vi "电导率电极校准.vi"() -> ()   [LabVIEW 2016, in "斯坦道多参数.lvlib"]
uses:
  <vilib>/Utility/miscctls.llb/LVPointTypeDef.ctl
  <vilib>/Analysis/NI_AALBase.lvlib
  <vilib>/ptbypt/NI_PtbyPt.lvlib
panel:
  in  "刷新按钮":bool
  out "第二点信号值":dbl
  out "第一点信号值":dbl
  out "通讯状态":string
  out "盐度":dbl caption="盐度测量值" format="%#.2f"
  out "温度":dbl format="%#.2f"
  out "当前信号值":dbl caption="信号值" format="%#.2f"
  in  "校准停止":bool
  in  "校准启动":bool
  out "波形图表":dbl(graph) caption="历史曲线"
  out "第二点校准值":dbl
  out "第一点校准值":dbl
  in  "校准模式":enum16{"两点校准", "单点校准"}(ring)=enum."单点校准"
  out "提示":string
  out "最小值":sgl format="%#.2f"
  out "最大值":sgl format="%#.2f"
  out "mean":dbl caption="均值" format="%#.2f"
  out "standard deviation":dbl caption="标准差" format="%#.2f"
  out "变异系数":dbl format="%#.6f"
  out "标液2":dbl
  out "标液1":dbl
  out "当前读取值":dbl caption="测量值" format="%#.2f"
  out "电极系数":dbl format="%#.6f"
  out "偏移值补偿":dbl caption="电导率偏移修正值" format="%#.2f"
  out "温度补偿系数":dbl format="%#.6f"
  # "电导率电极设定"
  # "ppt"
  # "请选择校准模式:"
  # "℃"
  # "μS/cm"
  # "cm"
  # "-1"
  # "%"
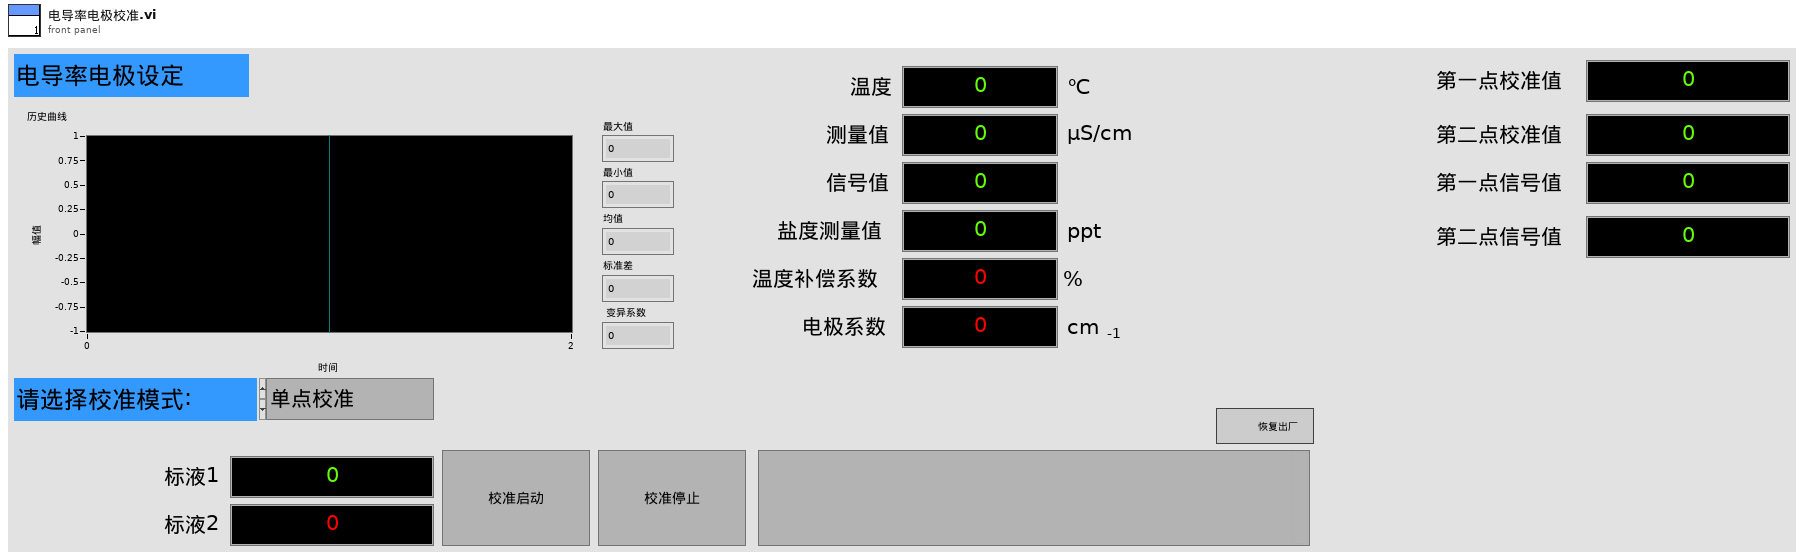
[diagram p1: front panel]
types:
  T1 = typedef "LVPointTypeDef.ctl" = cluster{"Horizontal":i16, "Vertical":i16}
  T2 = cluster{"电极状态标志":u16, "电极型号标志":u16, "电导率测量值":sgl, "温度测量值":sgl, "电导率信号值":sgl, "温度信号值":sgl, "温度补偿系数":sgl, "电导率偏移修正值":sgl, "温度偏移修正值":sgl, "手动温度补偿值":sgl, "电导率电极零点":sgl, "电导率电极斜率":sgl, "命令滤波设定":u16, "温度模式":enum16{"ATC", "MTC"}, "生产批次":u16, "电极序号":u16, "串口地址":u16, "串口波特率":enum16{"9600", "19200", "115200"}, "串口校验位":enum16{"NONE", "ODD", "EVEN"}, "串口停止位":enum16{"1bit", "2bit"}, "第一点标准值":sgl, "第二点标准值":sgl}
  T3 = enum8{"Enabled", "Disabled", "Disabled and Grayed Out"}
  T4 = cluster{"ph":bool, "DO":bool, "Cond":bool, "Turb":bool, "叶绿素a":bool, "藻密度":bool, "ORP":bool}
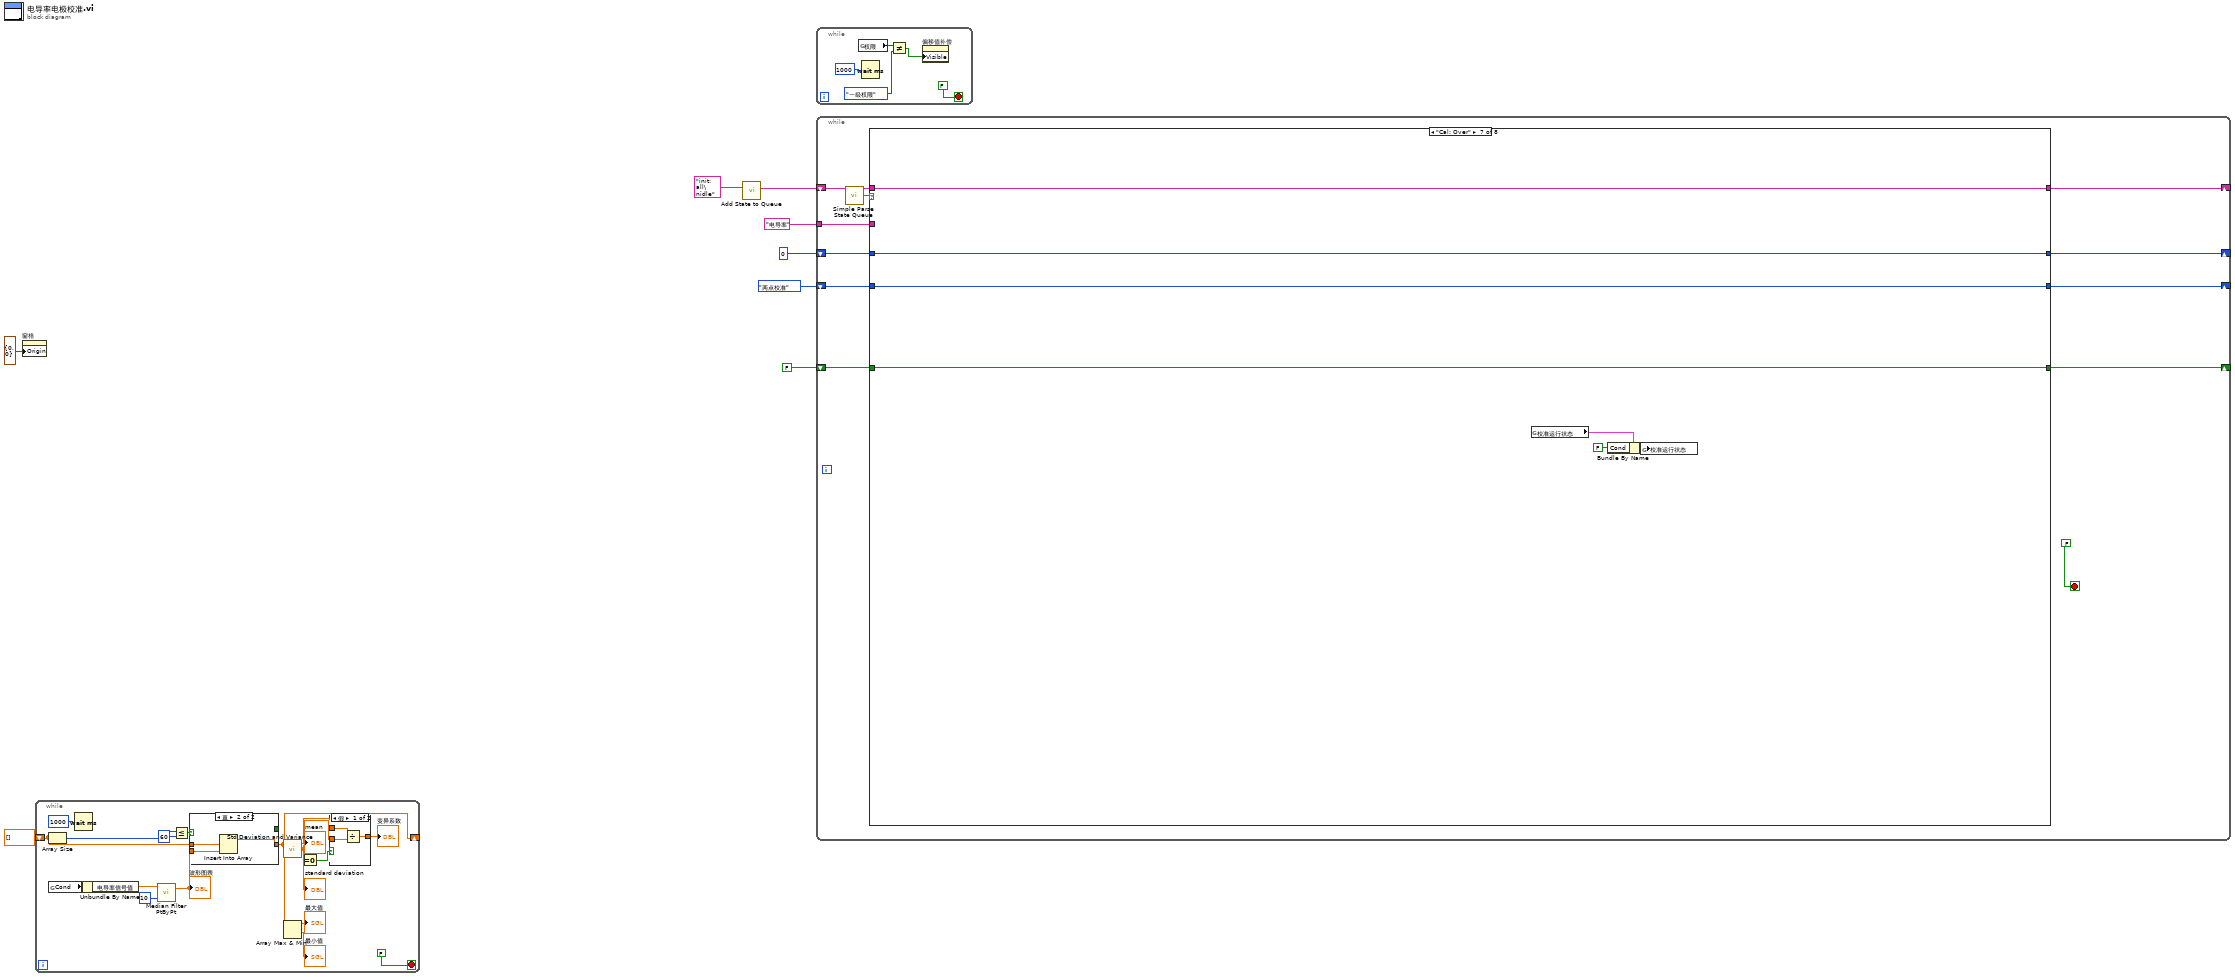
[diagram p0: block diagram]
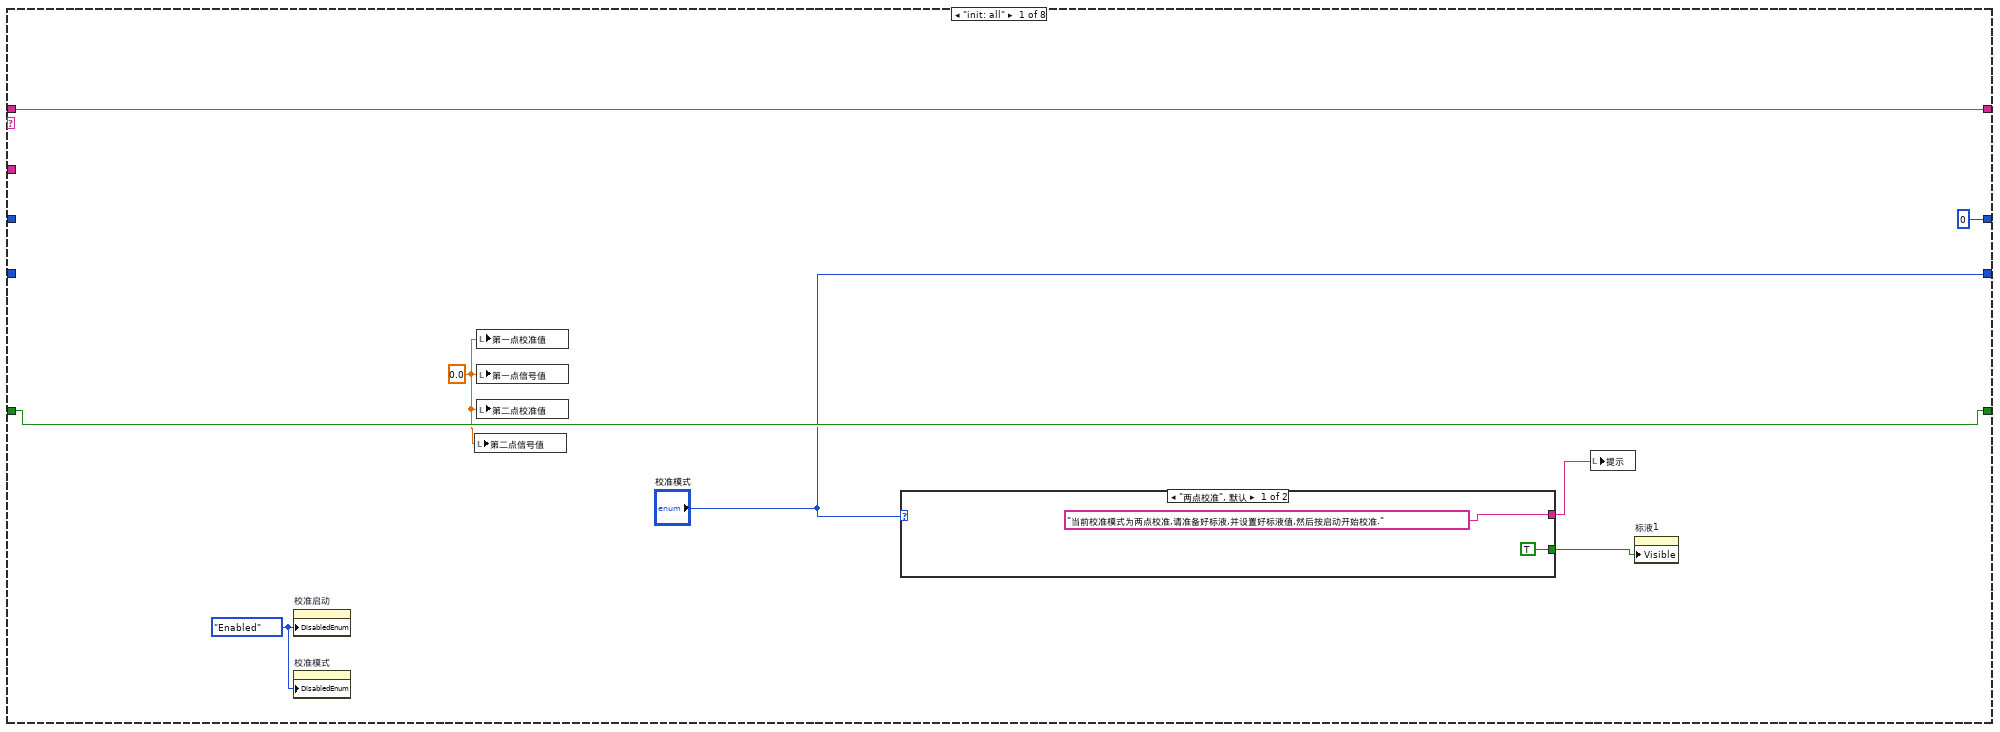
[diagram p2: hidden frame]
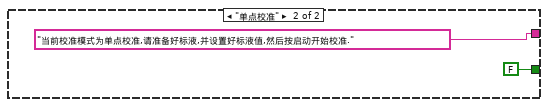
[diagram p3: hidden frame]
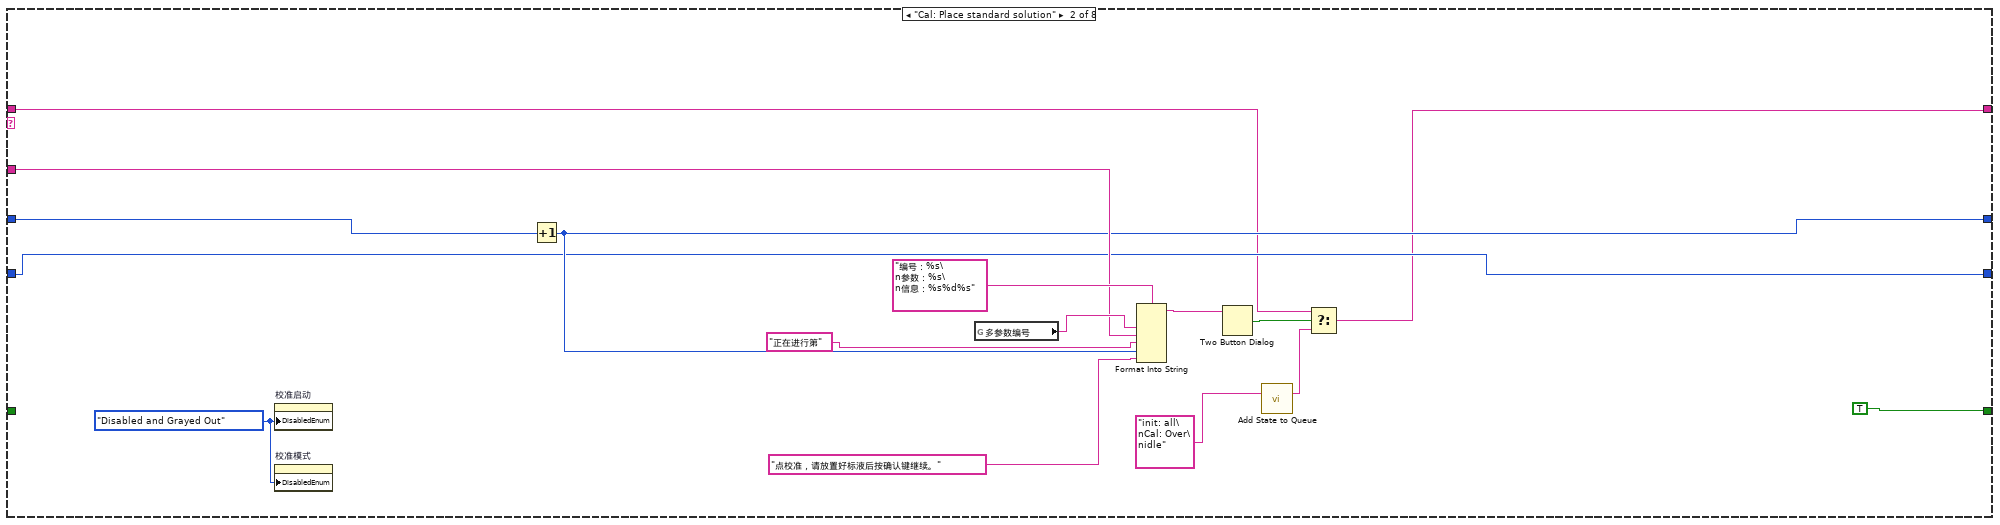
[diagram p4: hidden frame]
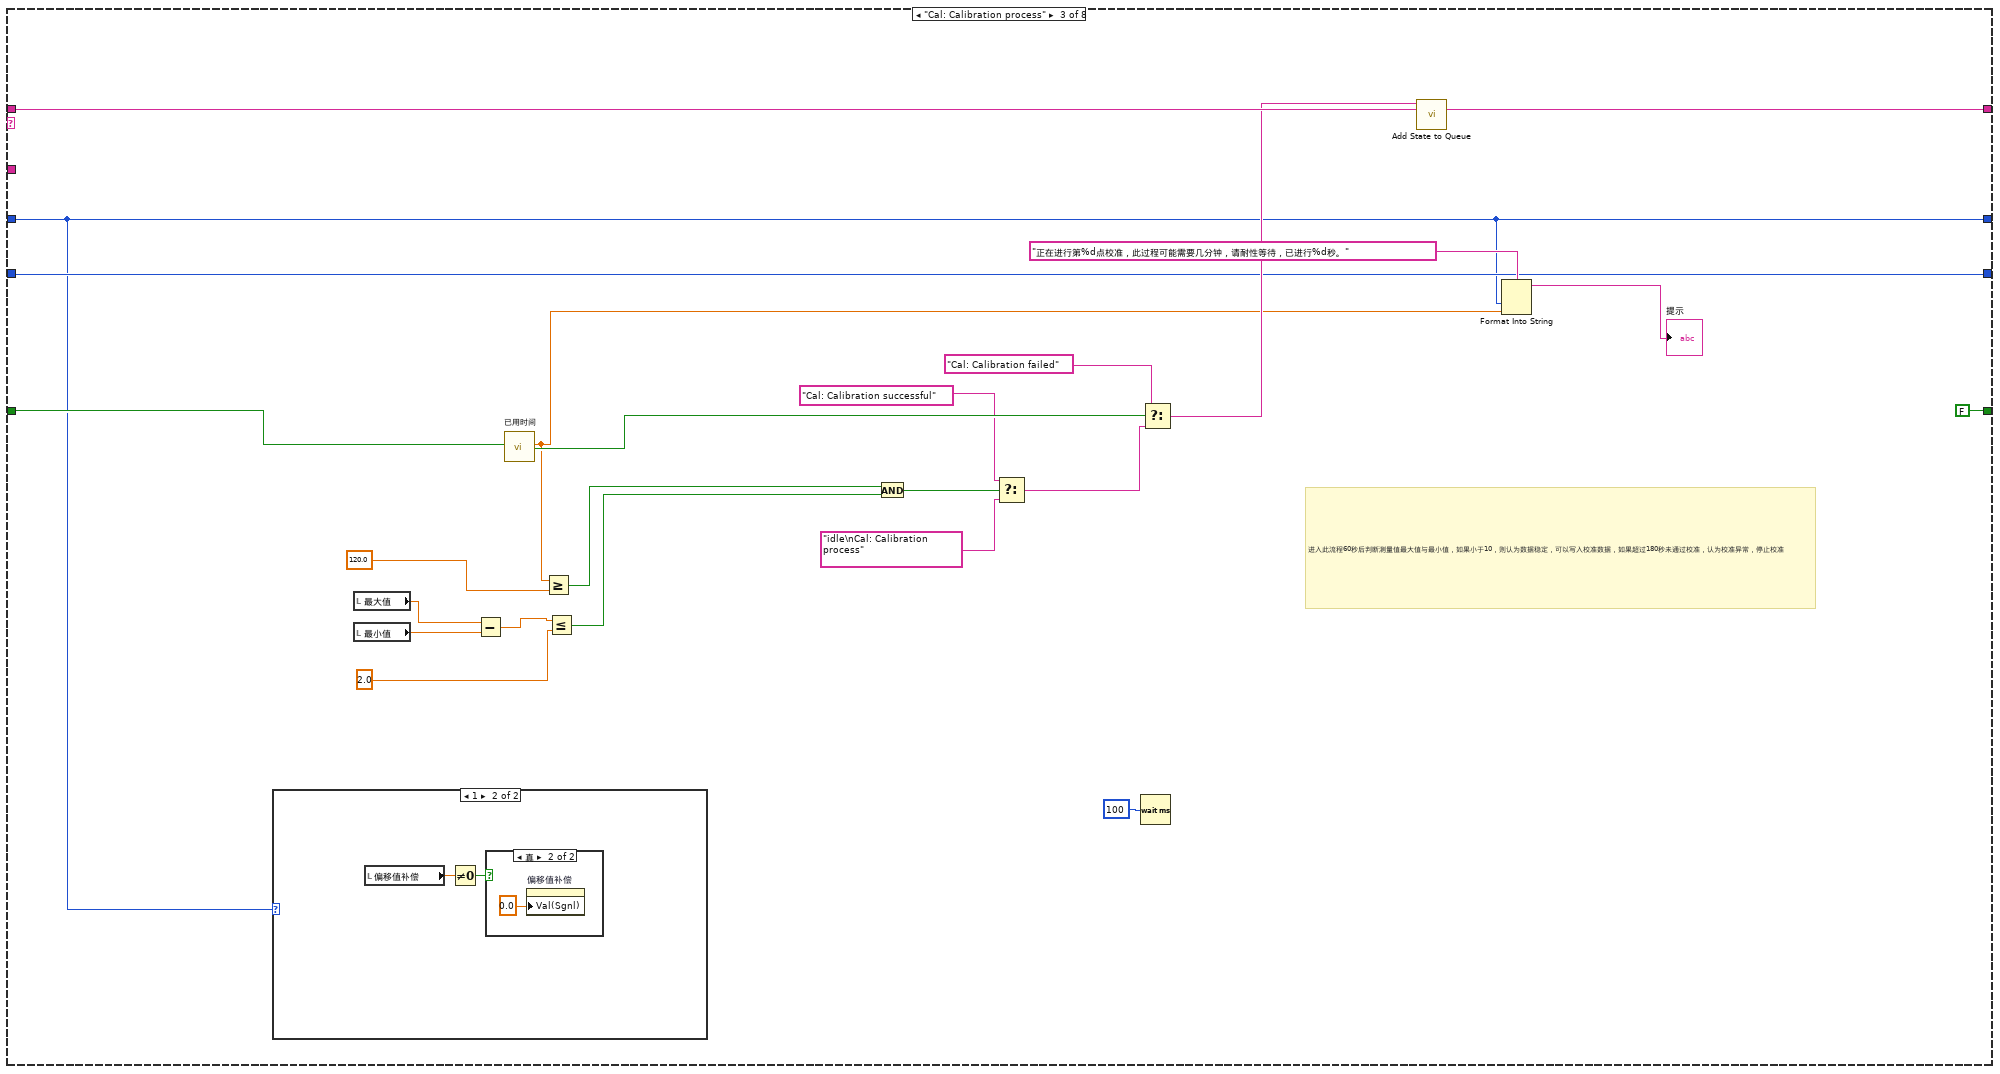
[diagram p5: hidden frame]
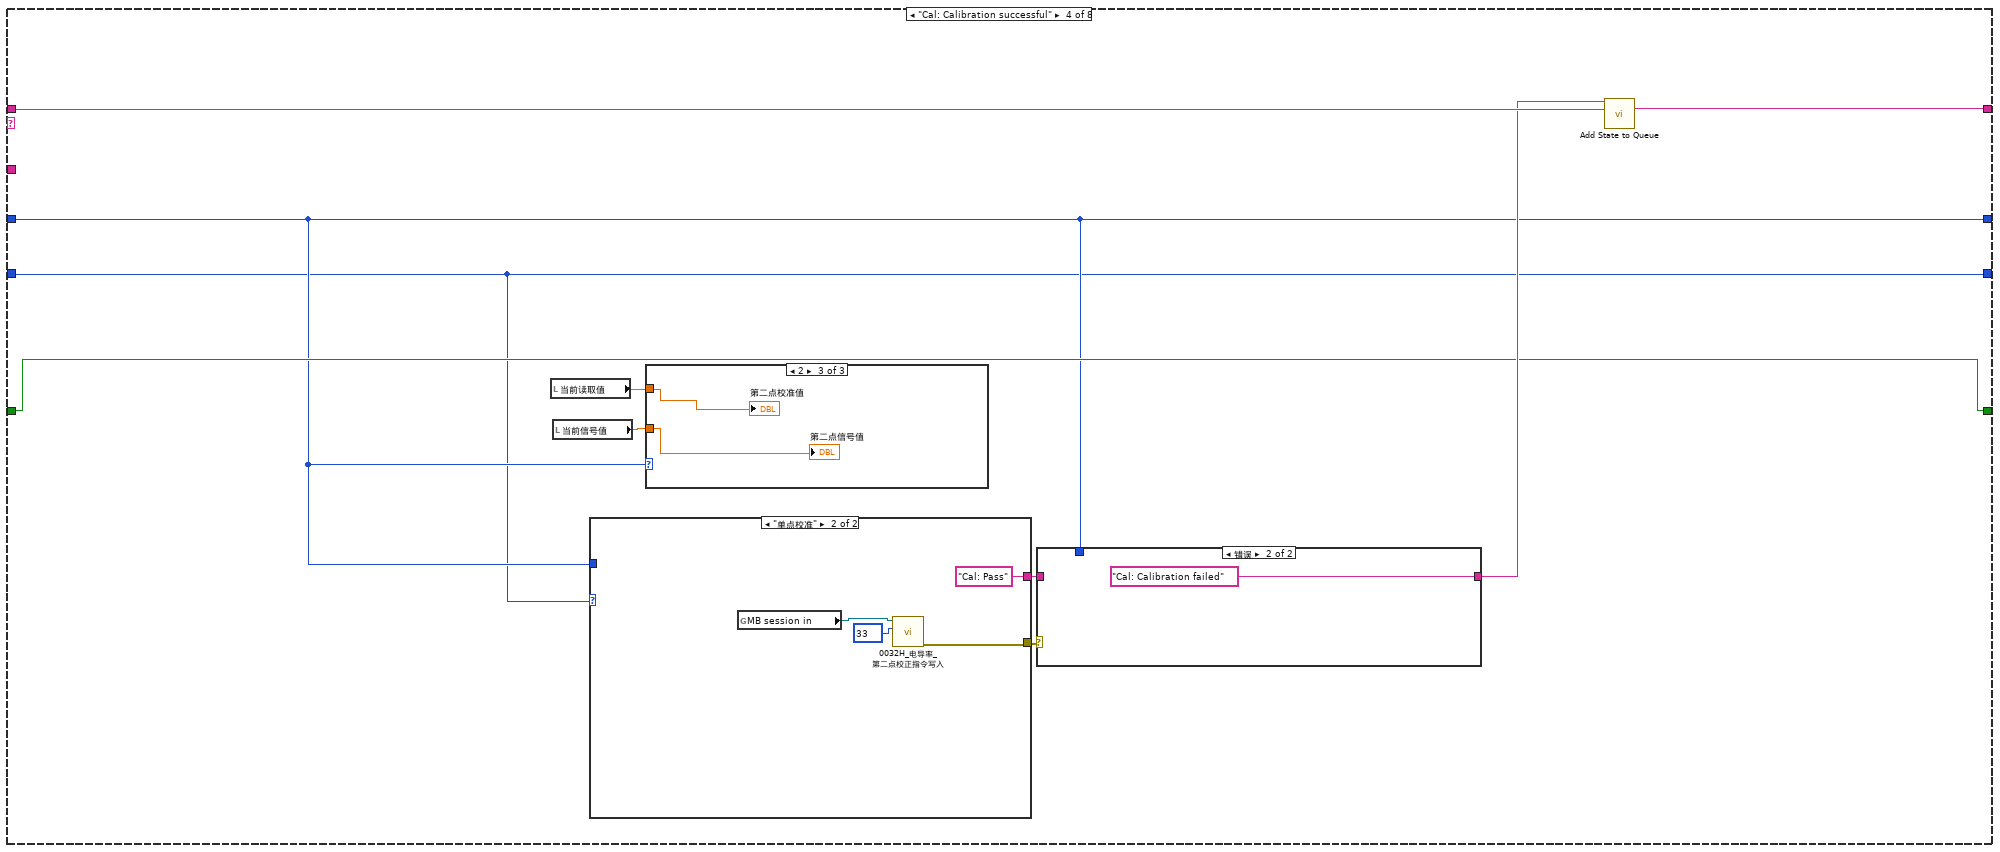
[diagram p8: hidden frame]
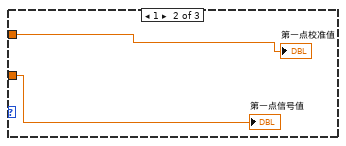
[diagram p10: hidden frame]
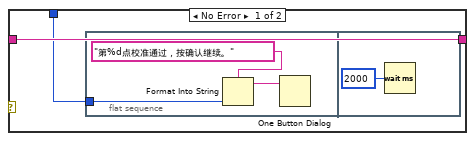
[diagram p11: hidden frame]
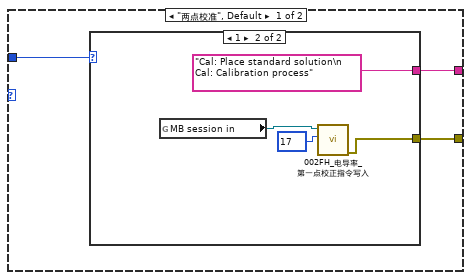
[diagram p12: hidden frame]
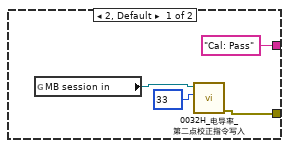
[diagram p13: hidden frame]
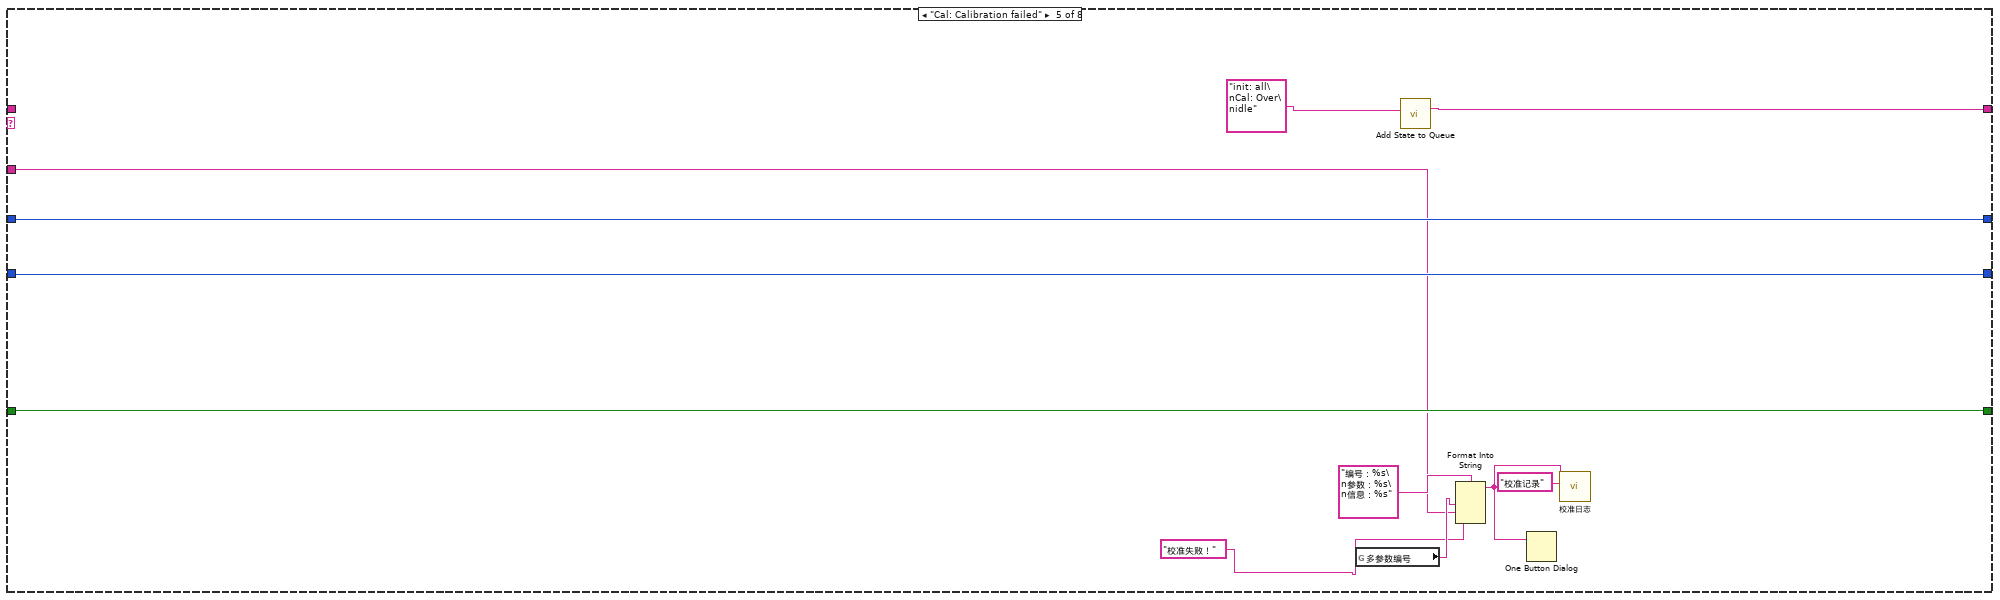
[diagram p14: hidden frame]
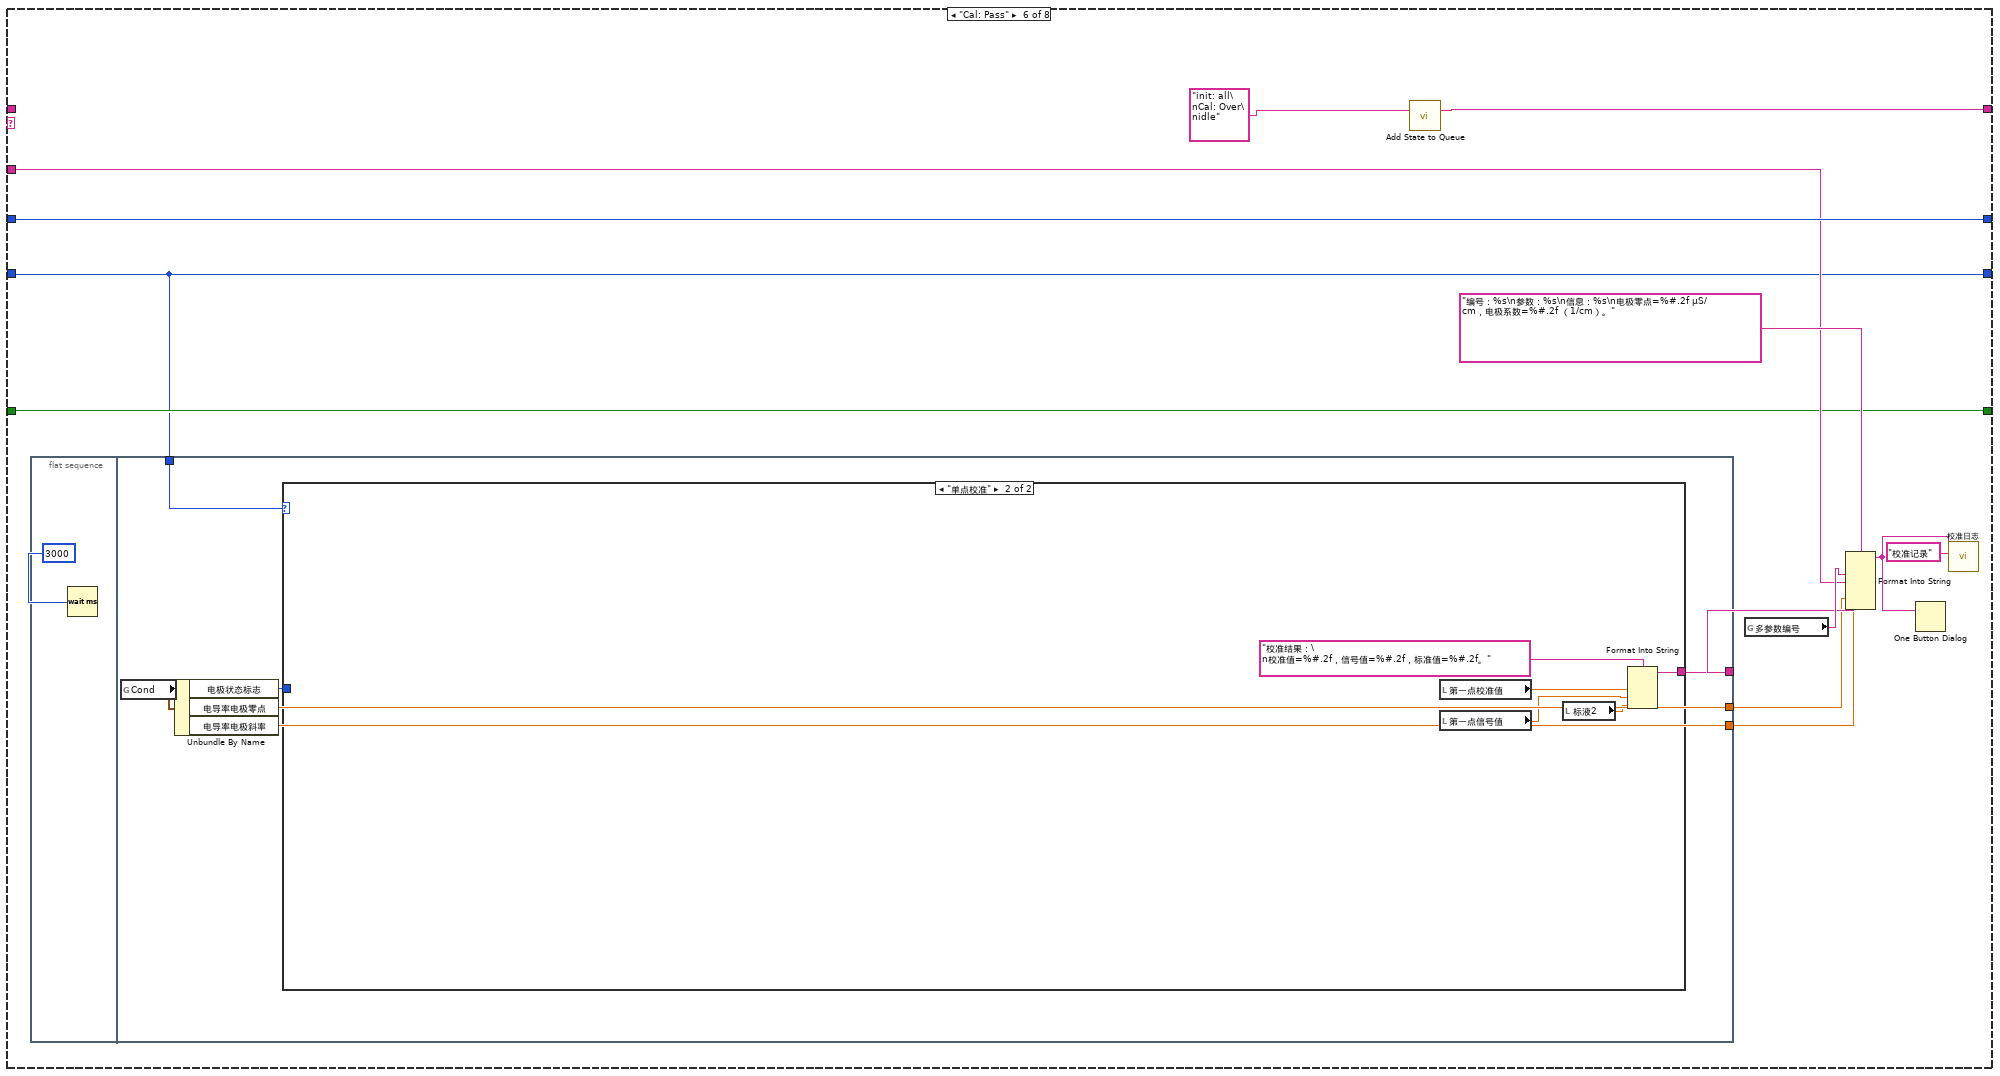
[diagram p15: hidden frame]
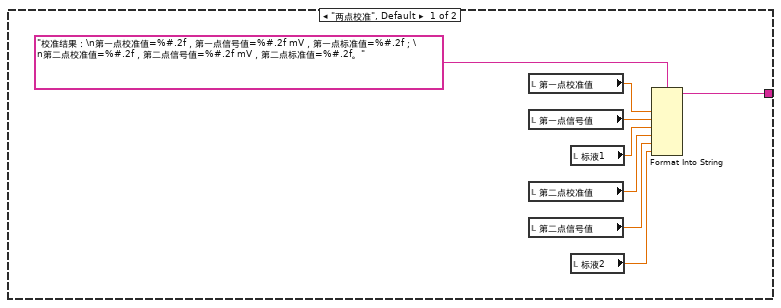
[diagram p16: hidden frame]
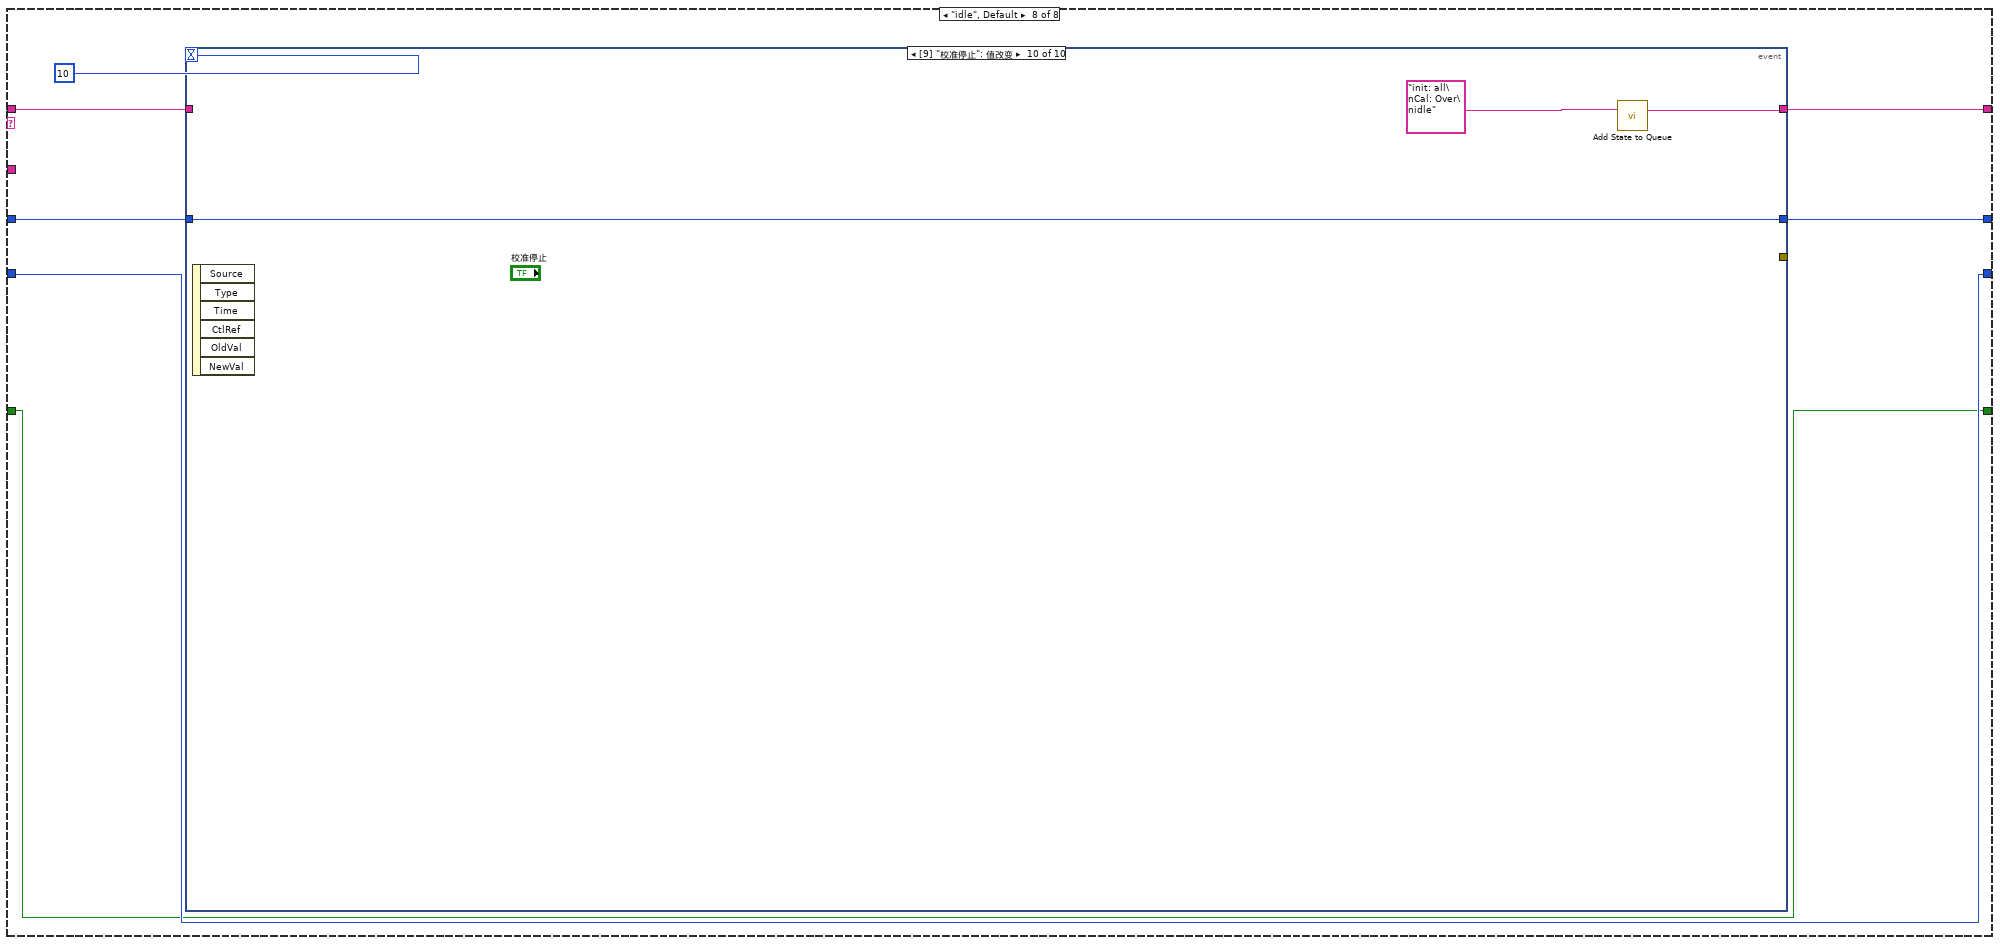
[diagram p17: hidden frame]
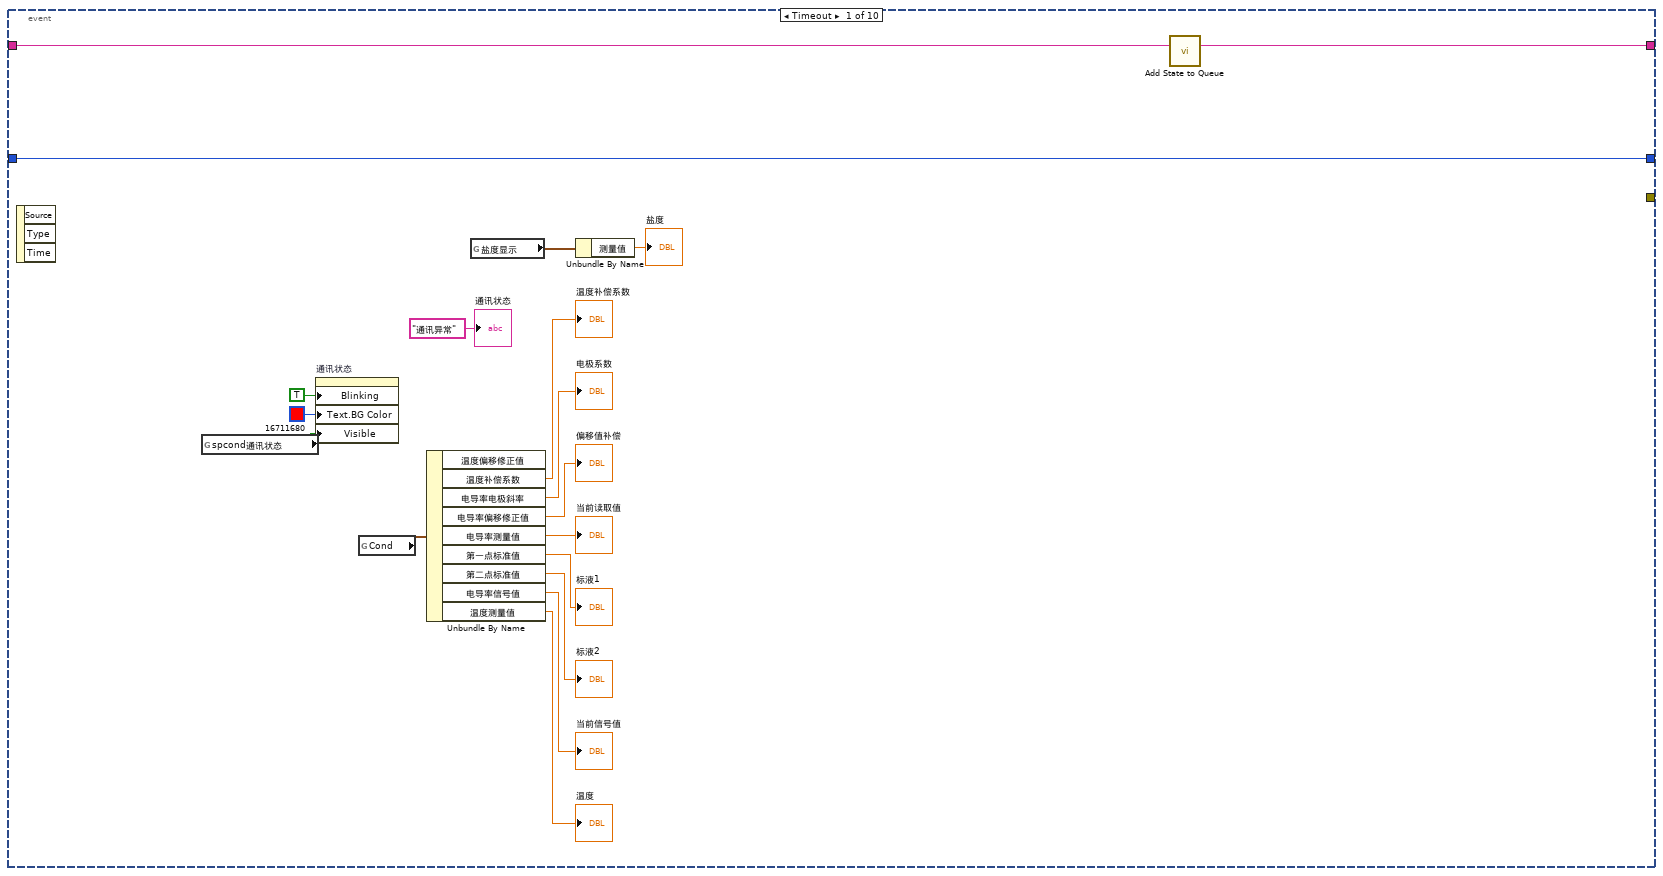
[diagram p18: hidden frame]
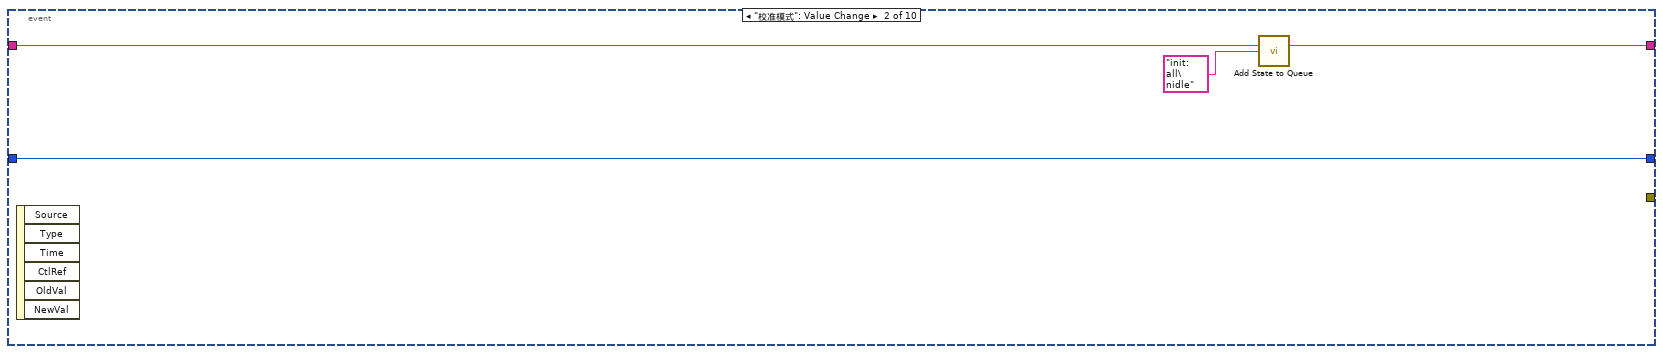
[diagram p19: hidden frame]
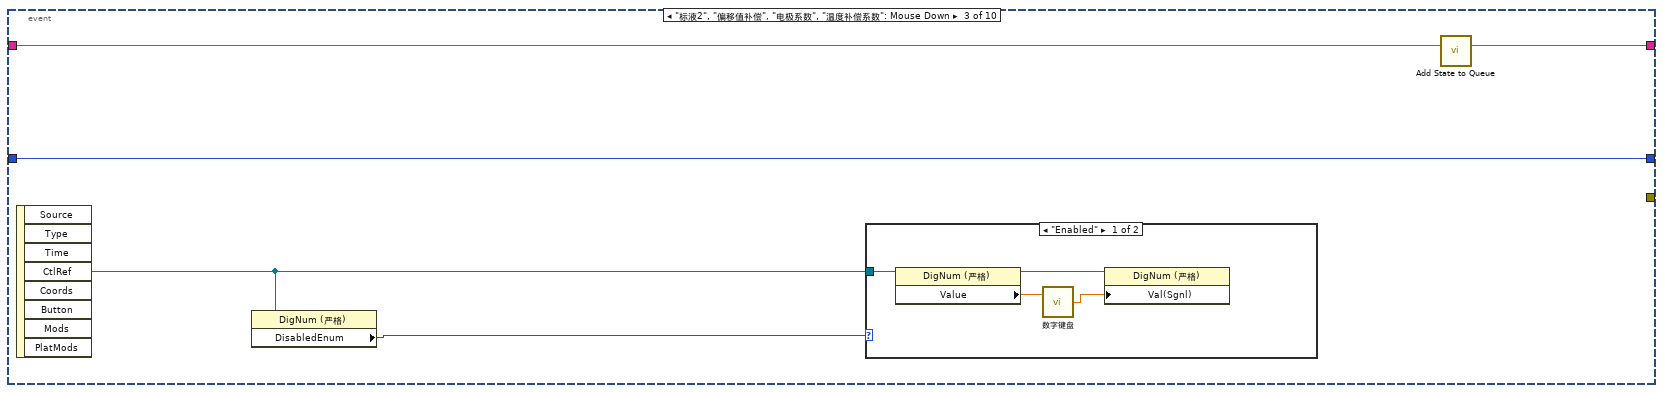
[diagram p20: hidden frame]
diagram:
  n1 = property on="窗格" class="Pane"("Origin"=T1 {"Horizontal"=0, "Vertical"=0} ("原点")) -> ()  [unwired: 2 in, 2 out]
  n2 = while {
    shift-right: [w14] -> _
    shift-left: sgl[] [] -> [w21]
    stop <- FALSE stop-if-true
    n3 = Array Size(array=w21) -> (size(s)=w23:i32)
    n4 = global read "国弘过程全局变量.vi" "Cond"() -> (w15:T2)
    n5 = Wait (ms)(milliseconds to wait=u32 1000 ("等待时间（毫秒）")) -> ()  [unwired: 1 out]
    n6 = Unbundle By Name(w15) -> ("电导率信号值"=w10:sgl)
    n7 = call <vilib>:"Median Filter PtByPt.vi"("rank"=10, "x"=w10) -> ("Filtered x"=w9:dbl)  [unwired: 2 in, 1 out]
    "波形图表" <- w9
    n8 = Less Or Equal?(x=w23, y=60) -> (x <= y?=w22:bool)
    n9 = case shown="真" w22 {
      tunnel: w21 -> [w34 w37]
      tunnel: w9 -> [w32 w36]
      tunnel: [w30 w35] -> w14
      tunnel: [TRUE _] -> _
      frame False {
        n10 = Replace Array Subset(array=w34, new element=w32) -> (w33:sgl[])  [unwired: 1 in]
        n11 = Rotate 1D Array(1:w33, 2:-1 ("n")) -> (0:w30:sgl[])
      }
      frame True {
        n12 = Insert Into Array(array=w37, new element=w36) -> (w35:sgl[])  [unwired: 1 in]
      }
    }
    n13 = call <vilib>:"Std Deviation and Variance.vi"("X"=w14) -> ("mean"=w19:dbl, "standard deviation"=w18:dbl)  [unwired: 1 in, 1 out]
    "mean" <- w19
    "standard deviation" <- w18
    n14 = Array Max & Min(array=w14) -> (max value=→"最大值":sgl, min value=→"最小值":sgl)  [unwired: 2 out]
    n15 = Equal To 0?(x=w19) -> (x = 0?=w20:bool)
    n16 = case shown="假" w20 {
      tunnel: w18 -> [w28 _]
      tunnel: [w27 _] -> w17
      tunnel: w19 -> [w26 _]
      frame False {
        n17 = Divide(x=w28, y=w26) -> (x/y=w27:dbl)
      }
      frame True {
      }
    }
    "变异系数" <- w17
  }
  n18 = call "Add State to Queue.vi"("State(s) In (\"\")"="init: all\nidle" ("State(s) In (\"\")")) -> ("States Out"=w5:string)  [unwired: 14 in]
  n19 = while {
    stop <- FALSE stop-if-true
    n20 = global read "多参数全局变量.vi" "权限"() -> (w41:enum16{"一级权限", "二级权限", "三级权限"})
    n21 = Wait (ms)(milliseconds to wait=u32 1000 ("等待时间（毫秒）")) -> ()  [unwired: 1 out]
    n22 = Not Equal?(x=w41, y=enum16{"一级权限", "二级权限", "三级权限"}."一级权限") -> (x != y?=w39:bool)
    n23 = property on="偏移值补偿" class="DigNum (严格)"("Visible"=w39) -> ()  [unwired: 2 in, 2 out]
  }
  n24 = while {
    shift-right: [w50] -> _
    shift-left: w5 -> [w54]
    shift-right: [w47] -> _
    shift-left: 0 -> [w49]
    tunnel: "电导率" ("State(s) In (\"\")") -> [w48]
    shift-right: [w45] -> _
    shift-left: enum16{"两点校准", "单点校准"}."两点校准" ("校准模式") -> [w46]
    shift-right: [w43] -> _
    shift-left: FALSE -> [w44]
    stop <- FALSE stop-if-true
    n25 = call "Simple Parse State Queue.vi"("State Queue"=w54) -> ("Remain States"=w51:string, "Next State"=w52:string)  [unwired: 13 in]
    n26 = case shown="\"Cal: Over\"" w52 {
      tunnel: w51 -> [w62 w70 w101 w117 _ _ w196 w203]
      tunnel: [w62 w69 w100 w116 w153 w160 w196 w202] -> w50
      tunnel: w49 -> [_ w78 w85 w111 w156 w169 w195 w200]
      tunnel: w48 -> [_ w79 _ _ w147 w165 _ _]
      tunnel: [0 w76 w85 w111 w156 w169 w195 w201] -> w47
      tunnel: w46 -> [_ w75 w86 w110 w155 w161 w194 w199]
      tunnel: ["校准模式" w75 w86 w110 w155 w161 w194 w199] -> w45
      tunnel: w44 -> [w59 _ w88 w112 w154 w164 w193 w197]
      tunnel: [w59 TRUE FALSE w112 w154 w164 w193 w197] -> w43
      frame "init: all" {
        w57 = T3."Enabled" ("禁用")
        w56 = 0.0 ("第一点校准值")
        n27 = property on="校准启动" class="Bool"("DisabledEnum"=w57) -> ()  [unwired: 2 in, 2 out]
        n28 = property on="校准模式" class="Enum (严格)"("DisabledEnum"=w57) -> ()  [unwired: 2 in, 2 out]
        n29 = local write "第二点信号值"(w56) -> ()
        n30 = local write "第一点校准值"(w56) -> ()
        n31 = local write "第一点信号值"(w56) -> ()
        n32 = local write "第二点校准值"(w56) -> ()
        n33 = case shown="\"两点校准\", 默认" "校准模式" {
          tunnel: ["当前校准模式为两点校准,请准备好标液,并设置好标液值,然后按启动开始校准." ("提示") "当前校准模式为单点校准,请准备好标液,并设置好标液值,然后按启动开始校准." ("提示")] -> w61
          tunnel: [TRUE ("可见") FALSE ("可见")] -> w55
          frame "两点校准", Default {
          }
          frame "单点校准" {
          }
        }
        n34 = local write "提示"(w61) -> ()
        n35 = property on="标液1" class="DigNum (严格)"("Visible"=w55) -> ()  [unwired: 2 in, 2 out]
      }
      frame "Cal: Place standard solution" {
        w68 = T3."Disabled and Grayed Out" ("禁用")
        n36 = property on="校准启动" class="Bool"("DisabledEnum"=w68) -> ()  [unwired: 2 in, 2 out]
        n37 = property on="校准模式" class="Enum (严格)"("DisabledEnum"=w68) -> ()  [unwired: 2 in, 2 out]
        n38 = Increment(x=w78) -> (x+1=w76:i32)
        n39 = global read "多参数全局变量.vi" "多参数编号"() -> (w81:string)
        n40 = Format Into String(format string="编号：%s\n参数：%s\n信息：%s%d%s" ("格式字符串"), w81, w79, "正在进行第" ("消息"), w76, "点校准，请放置好标液后按确认键继续。" ("消息")) -> (resulting string=w73:string)  [unwired: 2 in, 1 out]
        n41 = Two Button Dialog(message=w73) -> (T button?=w72:bool)  [unwired: 2 in]
        n42 = call "Add State to Queue.vi"("State(s) In (\"\")"="init: all\nCal: Over\nidle" ("State(s) In (\"\")")) -> ("States Out"=w71:string)  [unwired: 14 in]
        n43 = Select(t=w70, s=w72, f=w71) -> (s? t:f=w69:string)
      }
      frame "Cal: Calibration process" {
        # "进入此流程60秒后判断测量值最大值与最小值，如果小于10，则认为数据稳定，可以写入校准数据，如果超过180秒未通过校准，认为校准异常，停止校准"
        n44 = case shown="1" w85 {
          frame 0, Default {
          }
          frame 1 {
            n45 = local read "偏移值补偿"() -> (w107:dbl)
            n46 = Not Equal To 0?(x=w107) -> (x != 0?=w108:bool)
            n47 = case shown="真" w108 {
              frame False {
              }
              frame True {
                n48 = property on="偏移值补偿" class="DigNum (严格)"("Val(Sgnl)"=0.0 ("值(信号)")) -> ()  [unwired: 2 in, 2 out]
              }
            }
          }
        }
        n49 = local read "最大值"() -> (w105:sgl)
        n50 = local read "最小值"() -> (w104:sgl)
        n51 = Subtract(x=w105, y=w104) -> (x-y=w106:sgl)
        n52 = call "已用时间"("Reset"=w88) -> ("Elapsed Time (s)"=w84:dbl, "Time has Elapsed"=w102:bool)  [unwired: 11 in, 6 out]
        n53 = Greater Or Equal?(x=w84, y=120.0) -> (x >= y?=w97:bool)
        n54 = Less Or Equal?(x=w106, y=2.0) -> (x <= y?=w93:bool)
        n55 = And(x=w97, y=w93) -> (x .and. y?=w94:bool)
        n56 = Select(t="Cal: Calibration successful" ("State(s) In (\"\")"), s=w94, f="idle\nCal: Calibration process" ("State(s) In (\"\")")) -> (s? t:f=w92:string)
        n57 = Wait (ms)(milliseconds to wait=u32 100 ("等待时间（毫秒）")) -> ()  [unwired: 1 out]
        n58 = Select(t="Cal: Calibration failed" ("State(s) In (\"\")"), s=w102, f=w92) -> (s? t:f=w91:string)
        n59 = call "Add State to Queue.vi"("State(s) In Front (\"\")"=w91, "State(s) In (\"\")"=w101) -> ("States Out"=w100:string)  [unwired: 13 in]
        n60 = Format Into String(format string="正在进行第%d点校准，此过程可能需要几分钟，请耐性等待，已进行%d秒。" ("格式字符串"), w85, w84) -> (resulting string=→"提示":string)  [unwired: 2 in, 1 out]
      }
      frame "Cal: Calibration successful" {
        n61 = local read "当前读取值"() -> (w113:dbl)
        n62 = local read "当前信号值"() -> (w114:dbl)
        n63 = case shown="\"单点校准\"" w110 {
          tunnel: [w133 w142] -> w119
          tunnel: [w132 "Cal: Pass" ("State(s) In (\"\")")] -> w118
          tunnel: w111 -> [w131 _]
          frame "两点校准", Default {
            n64 = case shown="1" w131 {
              tunnel: [w134 w138] -> w133
              tunnel: ["Cal: Pass" ("State(s) In (\"\")") "Cal: Place standard solution\n Cal: Calibration process" ("State(s) In (\"\")")] -> w132
              frame 2, Default {
                n65 = global read "多参数全局变量.vi" "MB session in"() -> (w136:refnum<class "MB_Master.lvclass">)
                n66 = call "0032H_电导率_第二点校正指令写入.vi"("数值"=u16 33, "MB session in"=w136) -> ("error out"=w134:errorcluster)  [unwired: 8 in, 1 out]
              }
              frame 1 {
                n67 = global read "多参数全局变量.vi" "MB session in"() -> (w140:refnum<class "MB_Master.lvclass">)
                n68 = call "002FH_电导率_第一点校正指令写入.vi"("数值"=u16 17, "MB session in"=w140) -> ("error out"=w138:errorcluster)  [unwired: 8 in, 1 out]
              }
            }
          }
          frame "单点校准" {
            n69 = global read "多参数全局变量.vi" "MB session in"() -> (w144:refnum<class "MB_Master.lvclass">)
            n70 = call "0032H_电导率_第二点校正指令写入.vi"("数值"=u16 33, "MB session in"=w144) -> ("error out"=w142:errorcluster)  [unwired: 8 in, 1 out]
          }
        }
        n71 = case shown="2" w111 {
          tunnel: w114 -> [_ w121 w123]
          tunnel: w113 -> [_ w120 w122]
          frame 0, Default {
          }
          frame 1 {
            "第一点信号值" <- w121
            "第一点校准值" <- w120
          }
          frame 2 {
            "第二点信号值" <- w123
            "第二点校准值" <- w122
          }
        }
        n72 = case shown="错误" w119 {
          tunnel: w118 -> [w125 _]
          tunnel: [w125 "Cal: Calibration failed" ("State(s) In (\"\")")] -> w115
          tunnel: w111 -> [w124 _]
          frame No Error {
            n73 = flat-sequence {
              tunnel: w124 -> [w126]
              frame #0 {
                n74 = Format Into String(format string="第%d点校准通过，按确认继续。" ("格式字符串"), w126) -> (resulting string=w128:string)  [unwired: 2 in, 1 out]
                n75 = One Button Dialog(message=w128) -> ()  [unwired: 1 in, 1 out]
              }
              frame #1 {
                n76 = Wait (ms)(milliseconds to wait=u32 2000 ("等待时间（毫秒）")) -> ()  [unwired: 1 out]
              }
            }
          }
          frame Error {
          }
        }
        n77 = call "Add State to Queue.vi"("State(s) In Front (\"\")"=w115, "State(s) In (\"\")"=w117) -> ("States Out"=w116:string)  [unwired: 13 in]
      }
      frame "Cal: Calibration failed" {
        n78 = global read "多参数全局变量.vi" "多参数编号"() -> (w150:string)
        n79 = call "Add State to Queue.vi"("State(s) In (\"\")"="init: all\nCal: Over\nidle" ("State(s) In (\"\")")) -> ("States Out"=w153:string)  [unwired: 14 in]
        n80 = Format Into String(format string="编号：%s\n参数：%s\n信息：%s" ("格式字符串"), w150, w147, "校准失败！" ("消息")) -> (resulting string=w149:string)  [unwired: 2 in, 1 out]
        n81 = One Button Dialog(message=w149) -> ()  [unwired: 1 in, 1 out]
        n82 = call "校准日志.vi"("table"="校准记录", "日志信息"=w149) -> ()  [unwired: 9 in, 1 out]
      }
      frame "Cal: Pass" {
        n83 = flat-sequence {
          tunnel: [w174] -> w162
          tunnel: w161 -> [w173]
          tunnel: [w172] -> w159
          tunnel: [w171] -> w158
          frame #0 {
            n84 = Wait (ms)(milliseconds to wait=u32 3000 ("等待时间（毫秒）")) -> ()  [unwired: 1 out]
          }
          frame #1 {
            n85 = global read "国弘过程全局变量.vi" "Cond"() -> (w175:T2)
            n86 = Unbundle By Name(w175) -> ("电极状态标志"=w176:u16, "电导率电极零点"=w172:sgl, "电导率电极斜率"=w171:sgl)
            n87 = case shown="\"单点校准\"" w173 {
              tunnel: [w184 w189] -> w174
              tunnel: w176 -> [_ _]
              frame "两点校准", Default {
                n88 = local read "第一点校准值"() -> (w182:dbl)
                n89 = local read "第一点信号值"() -> (w183:dbl)
                n90 = local read "第二点校准值"() -> (w179:dbl)
                n91 = local read "第二点信号值"() -> (w178:dbl)
                n92 = local read "标液1"() -> (w180:dbl)
                n93 = local read "标液2"() -> (w177:dbl)
                n94 = Format Into String(format string="校准结果：\n第一点校准值=%#.2f，第一点信号值=%#.2f mV，第一点标准值=%#.2f；\n第二点校准值=%#.2f，第二点信号值=%#.2f mV，第二点标准值=%#.2f。" ("提示"), w182, w183, w180, w179, w178, w177) -> (resulting string=w184:string)  [unwired: 2 in, 1 out]
              }
              frame "单点校准" {
                n95 = local read "第一点校准值"() -> (w188:dbl)
                n96 = local read "第一点信号值"() -> (w186:dbl)
                n97 = local read "标液2"() -> (w185:dbl)
                n98 = Format Into String(format string="校准结果：\n校准值=%#.2f，信号值=%#.2f，标准值=%#.2f。" ("提示"), w188, w186, w185) -> (resulting string=w189:string)  [unwired: 2 in, 1 out]
              }
            }
          }
        }
        n99 = call "Add State to Queue.vi"("State(s) In (\"\")"="init: all\nCal: Over\nidle" ("State(s) In (\"\")")) -> ("States Out"=w160:string)  [unwired: 14 in]
        n100 = global read "多参数全局变量.vi" "多参数编号"() -> (w166:string)
        n101 = Format Into String(format string="编号：%s\n参数：%s\n信息：%s\n电极零点=%#.2f μS/cm，电极系数=%#.2f （1/cm）。" ("格式字符串"), w166, w165, w162, w159, w158) -> (resulting string=w163:string)  [unwired: 2 in, 1 out]
        n102 = One Button Dialog(message=w163) -> ()  [unwired: 1 in, 1 out]
        n103 = call "校准日志.vi"("table"="校准记录", "日志信息"=w163) -> ()  [unwired: 9 in, 1 out]
      }
      frame "Cal: Over" {
        n104 = global read "多参数全局变量.vi" "校准运行状态"() -> (w191:T4)
        n105 = Bundle By Name(cluster=w191, "Cond"=FALSE) -> (w192:T4)
        n106 = global write "多参数全局变量.vi" "校准运行状态"(w192) -> ()
      }
      frame "idle", Default {
        n107 = event shown="[9] \"校准停止\": 值改变" {
          selector: _ -> [_ _ _ _ _ _ _ _ _ _]
          dyn-events: _ -> [_ _ _ _ _ _ _ _ _ _]
          timeout: 10 -> [_ _ _ _ _ _ _ _ _ _]
          tunnel: [_ _ _ w236 w244 w248 w253 _ _ _] -> _
          tunnel: w203 -> [w221 w225 w228 w235 w241 w252 w258 w263 w272 _]
          tunnel: [w220 w224 w229 w239 w242 w251 w257 w262 w271 w274] -> w202
          tunnel: [w219 w222 w230 w240 w243 w250 w256 w261 w269 w275] -> w201
          tunnel: w200 -> [w219 w222 w230 w240 w243 w250 w256 w261 w269 w275]
          event Timeout {
            n108 = event-data() -> ()  [unwired: 1 in, 3 out]
            n109 = global read "多参数全局变量.vi" "spcond通讯状态"() -> (w217:bool)
            n110 = property on="通讯状态" class="Str"("Blinking"=TRUE ("闪烁"), "Text.BG Color"=u32 16711680, "Visible"=w217) -> ()  [unwired: 2 in, 2 out]
            n111 = global read "国弘过程全局变量.vi" "Cond"() -> (w204:T2)
            n112 = Unbundle By Name(w204) -> ("温度补偿系数"=→"温度补偿系数":sgl, "电导率电极斜率"=→"电极系数":sgl, "电导率偏移修正值"=→"偏移值补偿":sgl, "电导率测量值"=→"当前读取值":sgl, "第一点标准值"=→"标液1":sgl, "第二点标准值"=→"标液2":sgl, "电导率信号值"=→"当前信号值":sgl, "温度测量值"=→"温度":sgl)  [unwired: 1 out]
            n113 = global read "多参数全局变量.vi" "盐度显示"() -> (w213:cluster{"温度测量值":sgl, "测量值":sgl, "温度偏移修正值":sgl})
            n114 = Unbundle By Name(w213) -> ("测量值"=→"盐度":sgl)
            n115 = call "Add State to Queue.vi"("State(s) In (\"\")"=w221) -> ("States Out"=w220:string)  [unwired: 14 in]
            "通讯状态" <- "通讯异常" ("当前串口")
          }
          event "校准模式": Value Change {
            n116 = event-data() -> ()  [unwired: 1 in, 6 out]
            n117 = call "Add State to Queue.vi"("State(s) In (\"\")"=w225, "State(s) At Back (\"\")"="init: all\nidle" ("State(s) In (\"\")")) -> ("States Out"=w224:string)  [unwired: 13 in]
          }
          event "标液2", "偏移值补偿", "电极系数", "温度补偿系数": Mouse Down {
            n118 = event-data() -> ("CtlRef"=w227:refnum<vi>)  [unwired: 1 in, 7 out]
            n119 = property class="DigNum (严格)"(reference=w227) -> ("DisabledEnum"=w226:T3)  [unwired: 1 in, 2 out]
            n120 = case shown="\"Enabled\"" w226 {
              tunnel: w227 -> [w234 _]
              frame "Enabled" {
                n121 = property class="DigNum (严格)"(reference=w234) -> (reference out=w231:refnum<vi>, "Value"=w232:dbl)  [unwired: 1 in, 1 out]
                n122 = call "数字键盘.vi"("OldNumber"=w232) -> ("NewNumber"=w233:dbl)  [unwired: 1 in]
                n123 = property class="DigNum (严格)"(reference=w231, "Val(Sgnl)"=w233) -> ()  [unwired: 1 in, 2 out]
              }
              frame "Disabled", Default {
              }
            }
            n124 = call "Add State to Queue.vi"("State(s) In (\"\")"=w228) -> ("States Out"=w229:string)  [unwired: 14 in]
          }
          event "标液2": Value Change {
            n125 = event-data() -> ("NewVal"=w237:dbl)  [unwired: 1 in, 5 out]
            n126 = global read "多参数全局变量.vi" "MB session in"() -> (w238:refnum<class "MB_Master.lvclass">)
            n127 = call "0033H_电导率_第二点标准值写入.vi"("数值"=w237, "MB session in"=w238) -> ("error out"=w236:errorcluster)  [unwired: 8 in, 1 out]
            n128 = call "Add State to Queue.vi"("State(s) In (\"\")"=w235) -> ("States Out"=w239:string)  [unwired: 14 in]
          }
          event "电极系数": Value Change {
            n129 = event-data() -> ("NewVal"=w245:dbl)  [unwired: 1 in, 5 out]
            n130 = global read "多参数全局变量.vi" "MB session in"() -> (w246:refnum<class "MB_Master.lvclass">)
            n131 = call "0014H_电导率_电极系数写入.vi"("数值"=w245, "MB session in"=w246) -> ("error out"=w244:errorcluster)  [unwired: 8 in, 1 out]
            n132 = call "Add State to Queue.vi"("State(s) In (\"\")"=w241) -> ("States Out"=w242:string)  [unwired: 14 in]
          }
          event "偏移值补偿": Value Change {
            n133 = event-data() -> ("NewVal"=w247:dbl)  [unwired: 1 in, 5 out]
            n134 = global read "多参数全局变量.vi" "MB session in"() -> (w249:refnum<class "MB_Master.lvclass">)
            n135 = call "000CH_电导率_电导率偏移修正值写入.vi"("数值"=w247, "MB session in"=w249) -> ("error out"=w248:errorcluster)  [unwired: 8 in, 1 out]
            n136 = call "Add State to Queue.vi"("State(s) In (\"\")"=w252) -> ("States Out"=w251:string)  [unwired: 14 in]
          }
          event "温度补偿系数": Value Change {
            n137 = event-data() -> ("NewVal"=w254:dbl)  [unwired: 1 in, 5 out]
            n138 = global read "多参数全局变量.vi" "MB session in"() -> (w255:refnum<class "MB_Master.lvclass">)
            n139 = call "000AH_电导率_温度补偿系数写入.vi"("数值"=w254, "MB session in"=w255) -> ("error out"=w253:errorcluster)  [unwired: 8 in, 1 out]
            n140 = call "Add State to Queue.vi"("State(s) In (\"\")"=w258) -> ("States Out"=w257:string)  [unwired: 14 in]
          }
          event "刷新按钮": Value Change {
            n141 = event-data() -> ()  [unwired: 1 in, 6 out]
            n142 = call "Add State to Queue.vi"("State(s) In (\"\")"=w263) -> ("States Out"=w262:string)  [unwired: 14 in]
            n143 = Two Button Dialog(message="请再次确实是否恢复出厂设置！" ("消息")) -> (T button?=w260:bool)  [unwired: 2 in]
            n144 = case shown="真" w260 {
              frame False {
              }
              frame True {
                w264 = u16 33 items=["Factory Reset"=33] ("数值")
                n145 = global read "多参数全局变量.vi" "MB session in"() -> (w265:refnum<class "MB_Master.lvclass">)
                n146 = call "0026H_电导率_命令寄存器写入.vi"("数值"=w264, "MB session in"=w265) -> ()  [unwired: 8 in, 2 out]
              }
            }
          }
          event "校准启动": Value Change {
            n147 = event-data() -> ()  [unwired: 1 in, 6 out]
            n148 = global read "多参数全局变量.vi" "校准运行状态"() -> (w267:T4)
            n149 = Bundle By Name(cluster=w267, "Cond"=TRUE) -> (w268:T4)
            n150 = global write "多参数全局变量.vi" "校准运行状态"(w268) -> ()
            n151 = call "Add State to Queue.vi"("State(s) In (\"\")"=w272, "State(s) At Back (\"\")"="init: all\nCal: Place standard solution\n Cal: Calibration process\nidle" ("State(s) In (\"\")")) -> ("States Out"=w271:string)  [unwired: 13 in]
          }
          event "校准停止": Value Change {
            n152 = event-data() -> ()  [unwired: 1 in, 6 out]
            n153 = call "Add State to Queue.vi"("State(s) In (\"\")"="init: all\nCal: Over\nidle" ("State(s) In (\"\")")) -> ("States Out"=w274:string)  [unwired: 14 in]
          }
        }
      }
    }
  }
